vi "BetterErrorText.vi"(8 "error in (no error)":errorcluster, 11 "Python":T2) -> (2 "Disabled":T1(ring), 3 "Python out":T2)   [LabVIEW 2022 SP3]
uses:
  PythonCtrl.ctl
  Processors.ctl
  <vilib>/Platform/browser.llb/Open URL in Default Browser (string).vi
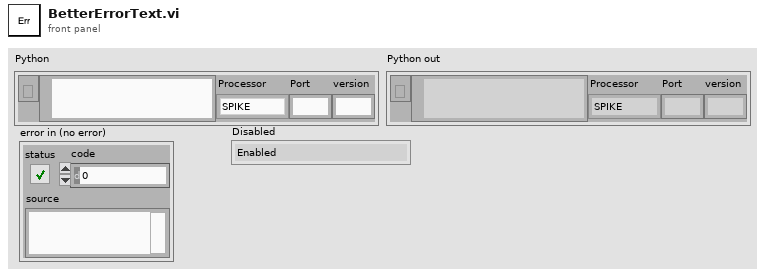
[diagram p1: front panel]
types:
  T1 = enum8{"Enabled", "Disabled", "Disabled and Grayed Out"}
  T2 = typedef "PythonCtrl.ctl" = cluster{"session":refnum<k35>, "PyPath":path, "Processor":T3, "Port":string, "version":string}
  T3 = typedef "Processors.ctl" = enum16{"SPIKE", "Pi", "Pi_ssh", "OpenMV", "Dunio"}
  T4 = enum16{"Left Button", "Center Button", "Right Button", "Window Close"}
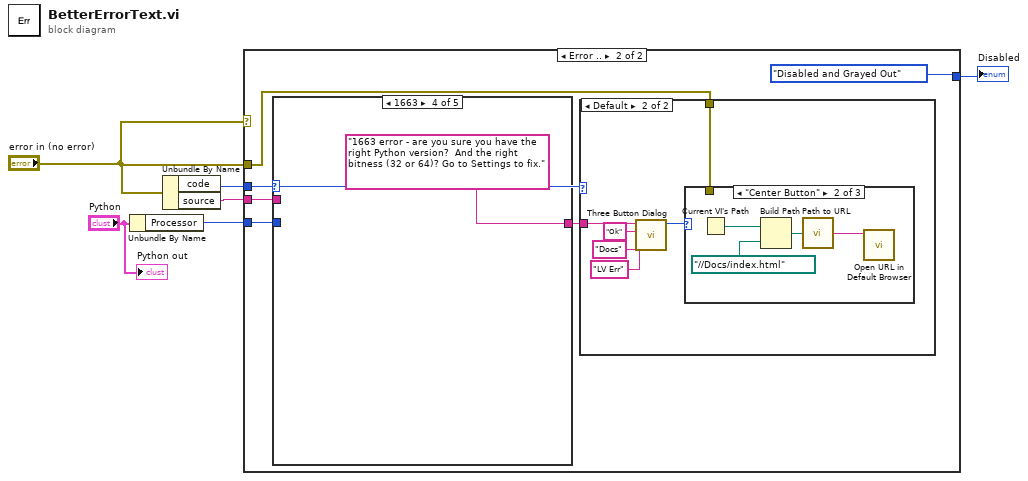
[diagram p0: block diagram]
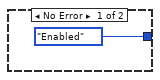
[diagram p2: hidden frame]
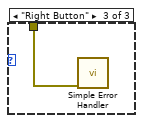
[diagram p5: hidden frame]
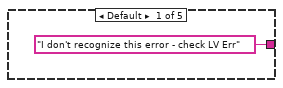
[diagram p6: hidden frame]
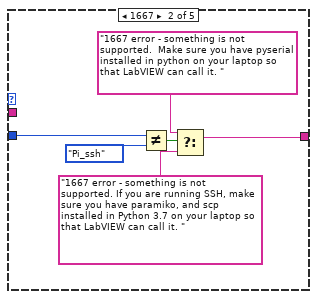
[diagram p7: hidden frame]
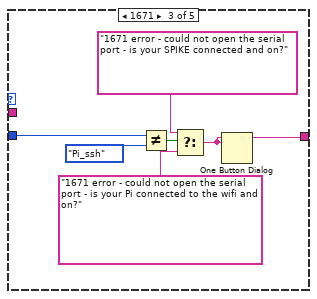
[diagram p8: hidden frame]
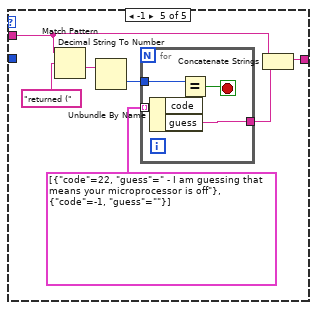
[diagram p9: hidden frame]
diagram:
  n1 = Unbundle By Name("Python") -> ("Processor"=w5:T3)
  n2 = Unbundle By Name("error in (no error)") -> ("code"=w3:i32, "source"=w4:string)
  n3 = case shown="Error .." "error in (no error)" {
    tunnel: w5 -> [_ w13]
    tunnel: w4 -> [_ w12]
    tunnel: "error in (no error)" -> [_ w10]
    tunnel: w3 -> [_ w9]
    tunnel: [T1."Enabled" ("Disabled") T1."Disabled and Grayed Out" ("Disabled")] -> w1
    frame No Error {
    }
    frame Error {
      n4 = case shown="1663" w9 {
        tunnel: w13 -> [_ w29 w35 _ _]
        tunnel: w12 -> [_ _ _ _ w43]
        tunnel: ["I don't recognize this error - check LV Err" ("message") w26 w32 "1663 error - are you sure you have the right Python version?  And the right bitness (32 or 64)? Go to Settings to fix." ("message") w41] -> w11
        frame Default {
        }
        frame 1667 {
          n5 = Not Equal?(x=w29, y=enum16{"SPIKE", "Pi", "Pi_ssh"}."Pi_ssh" ("Processor")) -> (x != y?=w31:bool)
          n6 = Select(t="1667 error - something is not supported.  Make sure you have pyserial installed in python on your laptop so that LabVIEW can call it. " ("message"), s=w31, f="1667 error - something is not supported. If you are running SSH, make sure you have paramiko, and scp installed in Python 3.7 on your laptop so that LabVIEW can call it. " ("message")) -> (s? t:f=w26:string)
        }
        frame 1671 {
          n7 = Not Equal?(x=w35, y=enum16{"SPIKE", "Pi", "Pi_ssh"}."Pi_ssh" ("Processor")) -> (x != y?=w37:bool)
          n8 = Select(t="1671 error - could not open the serial port - is your SPIKE connected and on?" ("message"), s=w37, f="1671 error - could not open the serial port - is your Pi connected to the wifi and on?" ("message")) -> (s? t:f=w32:string)
          n9 = One Button Dialog(message=w32) -> ()  [unwired: 1 in, 1 out]
        }
        frame 1663 {
        }
        frame -1 {
          n10 = Match Pattern(string=w43, regular expression="returned (") -> (after substring=w45:string)  [unwired: 1 in, 3 out]
          n11 = Decimal String To Number(string=w45) -> (number=w44:i32)  [unwired: 2 in, 1 out]
          n12 = for {
            tunnel: cluster{"code":i32, "guess":string}[] [{"code"=22, "guess"=" - I am guessing that means your microprocessor is off"}, {"code"=-1, "guess"=""}] -> [w50] mode=indexing
            tunnel: w44 -> [w49]
            tunnel: [w46] -> w42
            stop <- w47 stop-if-true
            n13 = Unbundle By Name(w50) -> ("code"=w48:i32, "guess"=w46:string)
            n14 = Equal?(x=w49, y=w48) -> (x = y?=w47:bool)
          }
          n15 = Concatenate Strings(w43, w42) -> (w41:string)
        }
      }
      n16 = case shown="Default" w9 {
        tunnel: w11 -> [_ w19]
        tunnel: w10 -> [_ w14]
        frame 0 {
        }
        frame Default {
          n17 = call <vilib>:"Three Button Dialog.vi"("Right Button Text (\"Cancel\")"="LV Err" ("Right Button Text (\"Cancel\")"), "Center Button Text (\"No\")"="Docs" ("Center Button Text (\"No\")"), "Left Button Text (\"Yes\")"="Ok" ("Left Button Text (\"Yes\")"), "message"=w19) -> ("Which Button?"=w15:T4)  [unwired: 7 in]
          n18 = case shown="\"Center Button\"" w15 {
            tunnel: w14 -> [_ _ w24]
            frame "Left Button", Default {
            }
            frame "Center Button" {
              n19 = Current VI's Path() -> (path=w23:path)
              n20 = Build Path(base path=w23, name or relative path=path "../../Docs/index.html") -> (appended path=w20:path)
              n21 = call <vilib>:"Path to URL.vi"("path"=w20) -> ("url"=w21:string)
              n22 = call-poly <vilib>:"Open URL in Default Browser.vi"("URL"=w21) -> ()  [unwired: 5 in, 2 out]
            }
            frame "Right Button" {
              n23 = call <vilib>:"Simple Error Handler.vi"("error in (no error)"=w24) -> ()  [unwired: 4 in, 5 out]
            }
          }
        }
      }
    }
  }
  "Disabled" <- w1
  "Python out" <- "Python"
